vi "First Matched Config File with Ext Options.vi"(4 "exts":string[](array[string]), 6 "Function Name":string="replace memory subs", 8 "Recursively(F)":bool, 11 "Searching Directory":path=path "") -> (3 "Config File":path)   [LabVIEW 2017]
doc: "Searches Searching Directory for the first file whose name matches Function Name with any of the extensions in exts. Set Recrusively(F) to search subfolders as well."
uses:
  4b0e83e5-5006-48cb-8f37-f4be335120c8.vi
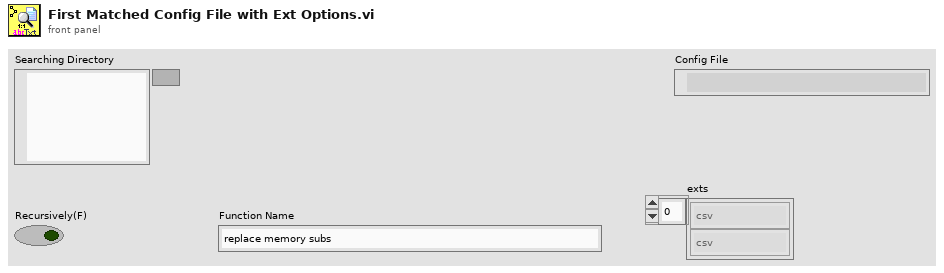
[diagram p1: front panel]
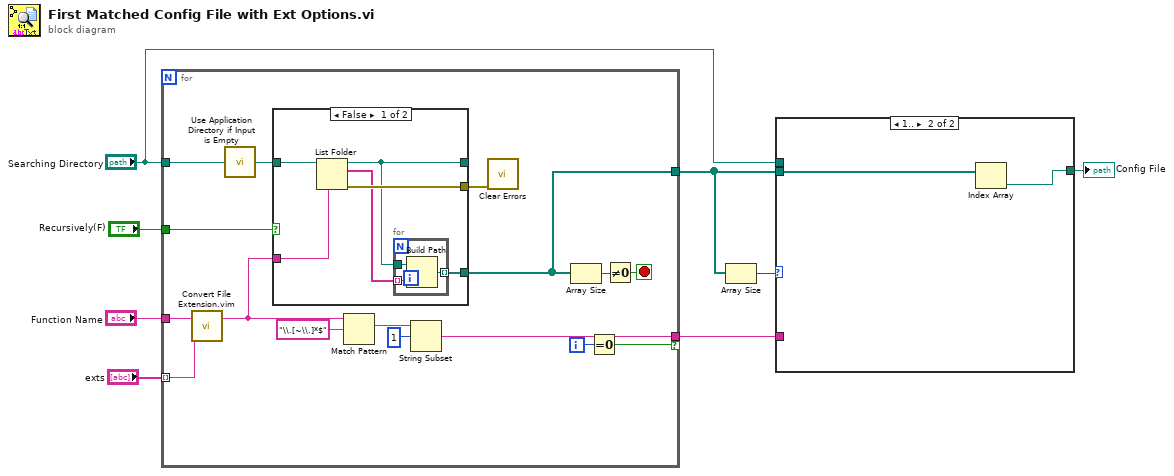
[diagram p0: block diagram]
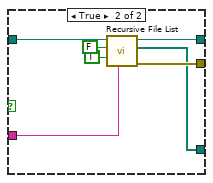
[diagram p2: hidden frame]
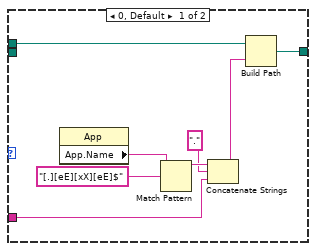
[diagram p3: hidden frame]
diagram:
  n1 = for {
    tunnel: "exts" -> [w24] mode=indexing
    tunnel: "Recursively(F)" -> [w23]
    tunnel: "Searching Directory" -> [w22]
    tunnel: "Function Name" -> [w21]
    tunnel: [w15] -> w5 if=w13
    tunnel: [w12] -> w4
    i -> [w14]
    stop <- w10 stop-if-true
    n2 = call "Convert File Extension.vim"("new ending (none)"=w24, "String/Path"=w21) -> ("new filename"=w9:string)  [unwired: 1 out]
    n3 = call "Use Application Directory if Input is Empty.vi"("Directory(Use Application Directory if Input is Empty)"=w22) -> ("Directory"=w16:path)
    n4 = case shown="False" w23 {
      tunnel: [w30 w38] -> w20
      tunnel: w9 -> [w28 w36]
      tunnel: w16 -> [w27 w39]
      tunnel: [w26 w37] -> w12
      tunnel: [w25 w40] -> _
      frame False {
        n5 = List Folder(path=w27, pattern=w28) -> (path out=w25:path, filenames=w29:string[], error out=w30:errorcluster)  [unwired: 2 in, 1 out]
        n6 = for {
          tunnel: w29 -> [w33] mode=indexing
          tunnel: [w32] -> w26 mode=indexing
          tunnel: w25 -> [w31]
          n7 = Build Path(base path=w31, name or relative path=w33) -> (appended path=w32:path)
        }
      }
      frame True {
        n8 = call <vilib>:"Recursive File List.vi"("pattern"=w36, "Continue Recursing on Error? (F)"=TRUE, "Treat LLBs as Folders?"=FALSE, "Folder Path"=w39) -> ("error out"=w38:errorcluster, "All Files in Dir"=w37:path[], "dup Folder Path"=w40:path)  [unwired: 3 in, 2 out]
      }
    }
    n9 = Match Pattern(string=w9, regular expression="\\.[~\\.]*$") -> (match substring=w17:string)  [unwired: 4 out]
    n10 = String Subset(string=w17, offset (0)=1) -> (substring=w15:string)  [unwired: 1 out]
    n11 = call <vilib>:"Clear Errors.vi"("error in (no error)"=w20) -> ()  [unwired: 5 in, 2 out]
    n12 = Array Size(array=w12) -> (size(s)=w11:i32)
    n13 = Equal To 0?(x=w14) -> (x = 0?=w13:bool)
    n14 = Not Equal To 0?(x=w11) -> (x != 0?=w10:bool)
  }
  n15 = Array Size(array=w4) -> (size(s)=w6:i32)
  n16 = case shown="1.." w6 {
    tunnel: w4 -> [_ w50]
    tunnel: "Searching Directory" -> [w48 _]
    tunnel: [w47 w49] -> w2
    tunnel: w5 -> [w41 _]
    frame 0, Default {
      n17 = property class="App"() -> ("App.Name"=w46:string)  [unwired: 2 in, 2 out]
      n18 = Match Pattern(string=w46, regular expression="[.][eE][xX][eE]$") -> (before substring=w44:string)  [unwired: 1 in, 3 out]
      n19 = Concatenate Strings(w44, "." ("string"), w41) -> (w43:string)
      n20 = Build Path(base path=w48, name or relative path=w43) -> (appended path=w47:path)
    }
    frame 1.. {
      n21 = Index Array(array=w50) -> (element=w49:path)  [unwired: 1 in]
    }
  }
  "Config File" <- w2
